vi "בדיקת צריכת זרם של סליל הפיקוד 5.vi"(7 "resultUserPrompt":bool, 8 "error":errorcluster, 10 "lines":tag="PXI1Slot8/port0/line1", 11 "Path for Log":path) -> (0 "error out":errorcluster, 2 "צריכת זרם בסליל בטווח כן/לא":bool, 3 "צריכת זרם בסליל":dbl format="%.4f")   [LabVIEW 2015]
uses:
  <vilib>/DAQmx/write.llb/DAQmx Write (Digital Bool 1Line 1Point).vi
  <vilib>/DAQmx/create/channels.llb/DAQmx Create Channel (DO-Digital Output).vi
  <vilib>/DAQmx/miscellaneous.llb/DAQmx Fill In Error Info.vi
panel:
  # "Right-Click to\nexplain error"
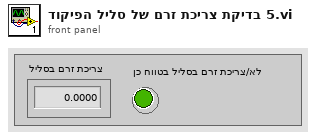
[diagram p1: front panel]
types:
  T1 = enum32{"Invalid", "Standard", "Closed", "Hidden", "Minimized", "Maximized"}
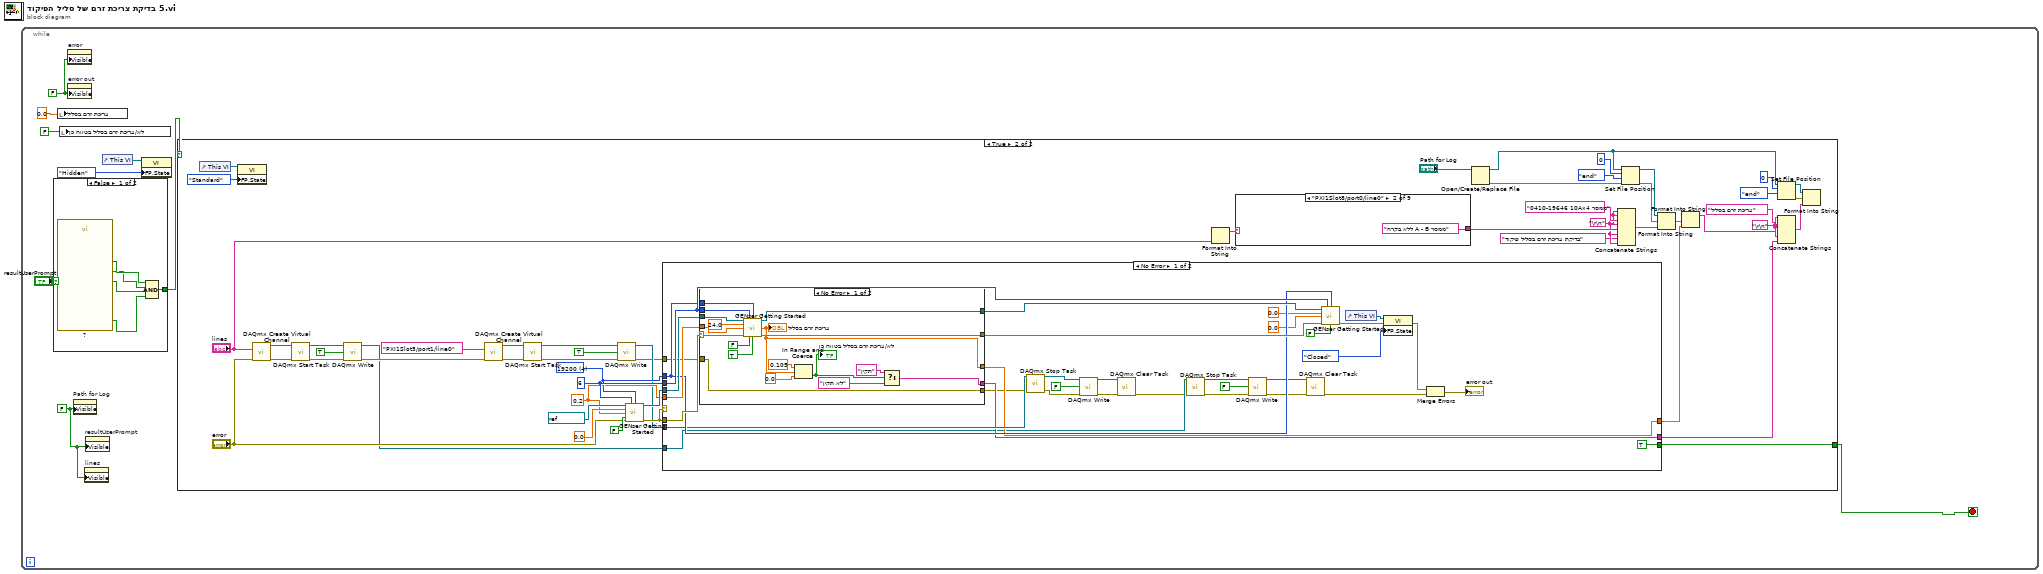
[diagram p0: block diagram]
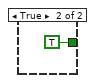
[diagram p2: hidden frame]
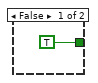
[diagram p3: hidden frame]
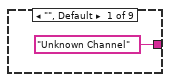
[diagram p4: hidden frame]
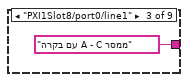
[diagram p5: hidden frame]
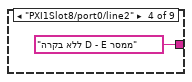
[diagram p6: hidden frame]
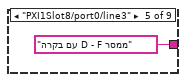
[diagram p7: hidden frame]
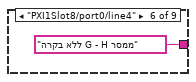
[diagram p8: hidden frame]
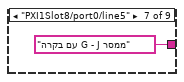
[diagram p9: hidden frame]
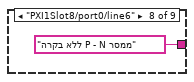
[diagram p10: hidden frame]
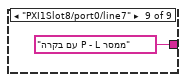
[diagram p11: hidden frame]
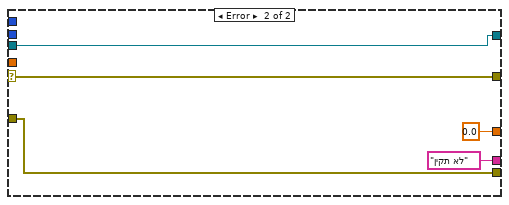
[diagram p12: hidden frame]
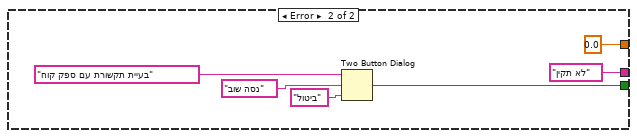
[diagram p13: hidden frame]
diagram:
  n1 = while {
    stop <- w1 stop-if-true
    w2 = FALSE ("Visible")
    w6 = FALSE ("Visible")
    n2 = case shown="False" "resultUserPrompt" {
      tunnel: [w14 TRUE] -> w9
      frame False {
        n3 = call "?"() -> ("הדקי הרב מודד"=w10:bool, "M מגע שלילי"=w11:bool, "K מגע חיובי"=w12:bool, "OK"=w13:bool)  [unwired: 15 in, 1 out]
        n4 = Compound Arithmetic op=AND(w13, w12, w11, w10) -> (w14:bool)
      }
      frame True {
      }
    }
    n5 = local write "צריכת זרם בסליל"(0.0 ("Output Current")) -> ()
    n6 = local write "צריכת זרם בסליל בטווח כן/לא"(FALSE ("In Range?")) -> ()
    n7 = property on="error" class="Clust (strict)"("Visible"=w6) -> ()  [unwired: 2 in, 2 out]
    n8 = property on="error out" class="Clust (strict)"("Visible"=w6) -> ()  [unwired: 2 in, 2 out]
    n9 = property on="Path for Log" class="Path"("Visible"=w2) -> ()  [unwired: 2 in, 2 out]
    n10 = property on="lines" class="DAQmxName"("Visible"=w2) -> ()  [unwired: 2 in, 2 out]
    n11 = property on="resultUserPrompt" class="Bool (strict)"("Visible"=w2) -> ()  [unwired: 2 in, 2 out]
    n12 = control-ref of="This VI"() -> (w5:refnum<vi>)
    n13 = property class="VI"(reference=w5, "FP.State"=T1."Hidden" ("Front Panel Window:State")) -> ()  [unwired: 1 in, 2 out]
    n14 = case shown="True" w9 {
      tunnel: [TRUE ("T button?") w61] -> w1
      frame False {
      }
      frame True {
        w23 = "\r\n"
        w43 = "\r\n"
        w60 = FALSE ("Output On (T)")
        w65 = u16 4 items=["1200", "2400", "4800", "9600", "19200"] ("BAUD")
        w66 = i16 6 ("GEN Addr")
        w62 = 0.2 ("Current Limit")
        n15 = control-ref of="This VI"() -> (w59:refnum<vi>)
        n16 = property class="VI"(reference=w59, "FP.State"=T1."Standard" ("Front Panel Window:State")) -> ()  [unwired: 1 in, 2 out]
        n17 = call-poly <vilib>:"DAQmx Create Virtual Channel.vi"("lines"="lines", "error in"="error") -> ("task out"=w35:refnum<k21>, "error out"=w36:errorcluster)  [unwired: 12 in]
        n18 = call <vilib>:"DAQmx Start Task.vi"("task/channels in"=w35, "error in"=w36) -> ("task out"=w38:refnum<k21>, "error out"=w37:errorcluster)  [unwired: 12 in]
        n19 = call-poly <vilib>:"DAQmx Write.vi"("task/channels in"=w38, "data"=TRUE, "error in"=w37) -> ("task out"=w32:refnum<k21>, "error out"=w33:errorcluster)  [unwired: 10 in, 1 out]
        n20 = call-poly <vilib>:"DAQmx Create Virtual Channel.vi"("lines"=tag "PXI1Slot5/port1/line0", "error in"=w33) -> ("task out"=w56:refnum<k21>, "error out"=w57:errorcluster)  [unwired: 12 in]
        n21 = call <vilib>:"DAQmx Start Task.vi"("task/channels in"=w56, "error in"=w57) -> ("task out"=w54:refnum<k21>, "error out"=w53:errorcluster)  [unwired: 12 in]
        n22 = call-poly <vilib>:"DAQmx Write.vi"("task/channels in"=w54, "data"=TRUE, "error in"=w53) -> ("task out"=w51:refnum<k21>, "error out"=w50:errorcluster)  [unwired: 10 in, 1 out]
        n23 = call "GENser Getting Started.vi"("VISA"=refnum<visa-resource-name> "COM6", "GEN Addr"=w66, "BAUD"=w65, "Voltage Limit"=0.0, "Current Limit"=w62, "error"="error", "Reset (T)"=w60, "Output On (T)"=w60) -> ("VISA out"=w67:refnum<visa-resource-name>, "error out"=w68:errorcluster)  [unwired: 4 in, 2 out]
        n24 = case shown="No Error" w68 {
          tunnel: w68 -> [w107 _]
          tunnel: w67 -> [w109 _]
          tunnel: w66 -> [w105 _]
          tunnel: w65 -> [w104 _]
          tunnel: w62 -> [w108 _]
          tunnel: [TRUE w137] -> w61
          tunnel: w51 -> [w103 _]
          tunnel: w50 -> [w99 _]
          tunnel: [w102 0.0 ("Output Current")] -> w49
          tunnel: [w101 "לא תקין"] -> w41
          tunnel: w32 -> [w100 _]
          frame No Error {
            n25 = case shown="No Error" w107 {
              selector: w107 -> [w118 w133]
              tunnel: [w124 w133] -> w110
              tunnel: w104 -> [w123 _]
              tunnel: w105 -> [w122 _]
              tunnel: w109 -> [w121 w134]
              tunnel: w108 -> [w120 _]
              tunnel: [w119 w134] -> w106
              tunnel: [w117 0.0 ("Output Current")] -> w102
              tunnel: [w113 "לא תקין"] -> w101
              tunnel: [w112 w130] -> w98
              tunnel: w99 -> [w112 w130]
              frame No Error {
                n26 = call "GENser Getting Started.vi"("VISA"=w121, "GEN Addr"=w122, "BAUD"=w123, "Voltage Limit"=24.0, "Current Limit"=w120, "error"=w118, "Reset (T)"=FALSE, "Output On (T)"=TRUE) -> ("VISA out"=w119:refnum<visa-resource-name>, "Output Current"=w117:dbl, "error out"=w124:errorcluster)  [unwired: 4 in, 1 out]
                "צריכת זרם בסליל" <- w117
                n27 = In Range and Coerce(upper limit=0.105, x=w117, lower limit=0.0) -> (In Range?=w114:bool)  [unwired: 1 out]
                "צריכת זרם בסליל בטווח כן/לא" <- w114
                n28 = Select(t="תקין", s=w114, f="לא תקין") -> (s? t:f=w113:string)
              }
              frame Error {
              }
            }
            n29 = call <vilib>:"DAQmx Stop Task.vi"("task/channels in"=w103, "error in"=w98) -> ("task out"=w91:refnum<k21>, "error out"=w90:errorcluster)  [unwired: 12 in]
            n30 = call-poly <vilib>:"DAQmx Write.vi"("task/channels in"=w91, "data"=FALSE, "error in"=w90) -> ("task out"=w89:refnum<k21>, "error out"=w88:errorcluster)  [unwired: 10 in, 1 out]
            n31 = call <vilib>:"DAQmx Clear Task.vi"("task in"=w89, "error in"=w88) -> ("error out"=w78:errorcluster)  [unwired: 13 in]
            n32 = call <vilib>:"DAQmx Stop Task.vi"("task/channels in"=w100, "error in"=w78) -> ("task out"=w84:refnum<k21>, "error out"=w82:errorcluster)  [unwired: 12 in]
            n33 = call-poly <vilib>:"DAQmx Write.vi"("task/channels in"=w84, "data"=FALSE, "error in"=w82) -> ("task out"=w81:refnum<k21>, "error out"=w80:errorcluster)  [unwired: 10 in, 1 out]
            n34 = call <vilib>:"DAQmx Clear Task.vi"("task in"=w81, "error in"=w80) -> ("error out"=w79:errorcluster)  [unwired: 13 in]
            n35 = call "GENser Getting Started.vi"("VISA"=w106, "GEN Addr"=w105, "BAUD"=w104, "Voltage Limit"=0.0, "Current Limit"=0.0, "error"=w110, "Output On (T)"=FALSE) -> ("error out"=w92:errorcluster)  [unwired: 5 in, 3 out]
            n36 = control-ref of="This VI"() -> (w94:refnum<vi>)
            n37 = property class="VI"(reference=w94, error in=w92, "FP.State"=T1."Closed" ("Front Panel Window:State")) -> (error out=w86:errorcluster)  [unwired: 1 out]
            n38 = Merge Errors(w86, w79) -> (→"error out":errorcluster)
          }
          frame Error {
            n39 = Two Button Dialog(message="בעיית תקשורת עם ספק קוח", 1:"ביטול" ("F button name (\"Cancel\")"), 2:"נסה שוב" ("T button name (\"OK\")")) -> (T button?=w137:bool)
          }
        }
        n40 = Format Into String("lines") -> (resulting string=w26:string)  [unwired: 3 in, 1 out]
        n41 = case shown="\"PXI1Slot8/port0/line0\"" w26 {
          tunnel: ["Unknown Channel" "ללא בקרה A - B ממסר" "עם בקרה A - C ממסר" "ללא בקרה D - E ממסר" "עם בקרה D - F ממסר" "ללא בקרה G - H ממסר" "עם בקרה G - J ממסר" "ללא בקרה P - N ממסר" "עם בקרה P - L ממסר"] -> w25
          frame "", Default {
          }
          frame "PXI1Slot8/port0/line0" {
          }
          frame "PXI1Slot8/port0/line1" {
          }
          frame "PXI1Slot8/port0/line2" {
          }
          frame "PXI1Slot8/port0/line3" {
          }
          frame "PXI1Slot8/port0/line4" {
          }
          frame "PXI1Slot8/port0/line5" {
          }
          frame "PXI1Slot8/port0/line6" {
          }
          frame "PXI1Slot8/port0/line7" {
          }
        }
        n42 = Open/Create/Replace File(file path (use dialog)="Path for Log") -> (refnum out=w18:refnum<file>, error out=w29:errorcluster)  [unwired: 5 in, 1 out]
        n43 = Concatenate Strings(w23, w23, "0410-19646 10Ax4 ממסר", w23, w25, w23, "בדיקת צריכת זרם בסליל פיקוד", w23) -> (w28:string)
        n44 = Set File Position(offset (in bytes) (0)=i64 0, refnum=w18, from (0:start)=enum16{"start", "end", "current"}."end", error in=w29) -> (refnum out=w27:refnum<file>, error out=w20:errorcluster)
        n45 = Format Into String(initial string=w27, error in=w20, w28) -> (error out=w19:errorcluster)  [unwired: 1 in, 1 out]
        n46 = Format Into String(error in=w19, w49) -> (resulting string=w40:string)  [unwired: 2 in, 1 out]
        n47 = Set File Position(offset (in bytes) (0)=i64 0, refnum=w18, from (0:start)=enum16{"start", "end", "current"}."end") -> (refnum out=w46:refnum<file>, error out=w47:errorcluster)  [unwired: 1 in]
        n48 = Concatenate Strings(w43, "צריכת זרם בסליל", w43, w40, w43, w41) -> (w48:string)
        n49 = Format Into String(initial string=w46, error in=w47, w48) -> ()  [unwired: 1 in, 2 out]
      }
    }
  }
